vi "14.Evd.5_Ask.4.vi"() -> ()   [LabVIEW 2025]
panel:
  in  "Ms Delay":u32=1000
  in  "Stop":bool
  out "B":bool
  out "A":bool
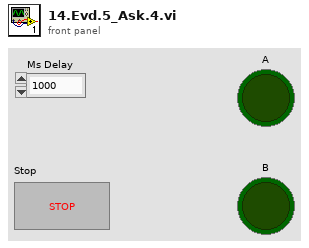
[diagram p1: front panel]
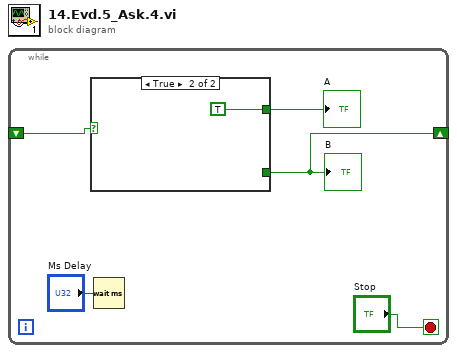
[diagram p0: block diagram]
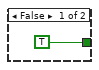
[diagram p2: hidden frame]
diagram:
  n1 = while {
    shift-right: [w1] -> _
    shift-left: _ -> [w4]
    stop <- "Stop" stop-if-true
    n2 = case shown="True" w4 {
      tunnel: [_ TRUE] -> w2
      tunnel: [TRUE _] -> w1
      frame False {
      }
      frame True {
      }
    }
    "A" <- w2
    "B" <- w1
    n3 = Wait (ms)(milliseconds to wait="Ms Delay") -> ()  [unwired: 1 out]
  }
